vi "file.tif.Write.vi"(7 "name":string, 8 "error in":errorcluster, 10 "u16 pixmap":u16[][](array[numeric]), 11 "path":path) -> (0 "error out":errorcluster)   [LabVIEW 2020]
uses:
  lib/fileIO.x64.dll
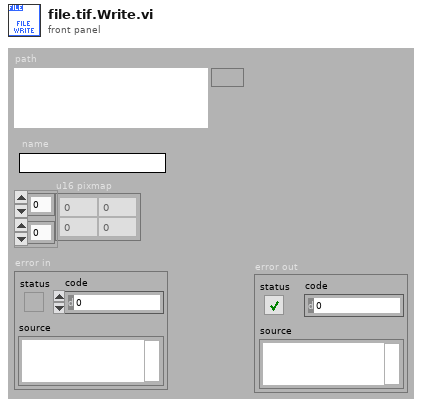
[diagram p1: front panel]
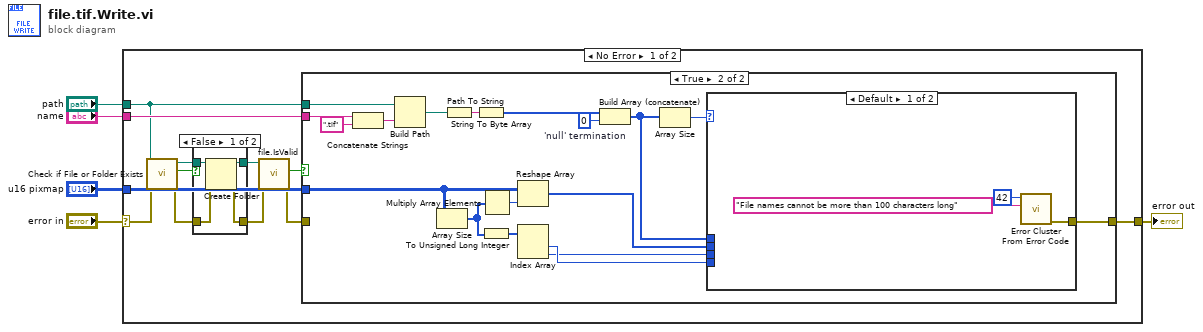
[diagram p0: block diagram]
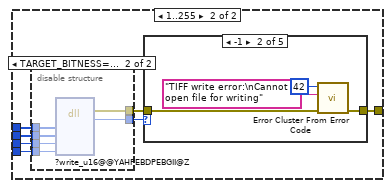
[diagram p3: hidden frame]
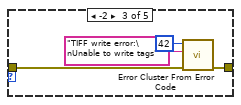
[diagram p5: hidden frame]
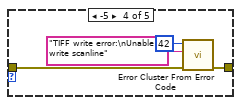
[diagram p6: hidden frame]
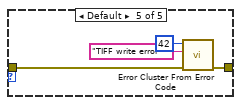
[diagram p7: hidden frame]
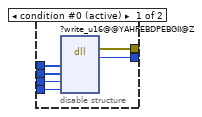
[diagram p8: hidden frame]
diagram:
  n1 = case shown="No Error" "error in" {
    selector: "error in" -> [w15 w82]
    tunnel: "path" -> [w6 _]
    tunnel: "u16 pixmap" -> [w17 _]
    tunnel: [w16 w82] -> w2
    tunnel: "name" -> [w9 _]
    frame No Error {
      n2 = call <vilib>:"Check if File or Folder Exists.vi"("error in (no error)"=w15, "path"=w6) -> ("error out"=w13:errorcluster, "file or folder exists?"=w11:bool, "dup path"=w7:path)  [unwired: 7 in]
      n3 = case shown="False" w11 {
        tunnel: w7 -> [w79 w80]
        tunnel: w13 -> [w78 w81]
        tunnel: [w77 w81] -> w12
        tunnel: [w76 w80] -> w8
        frame False {
          n4 = Create Folder(path (use dialog)=w79, error in=w78) -> (created path=w76:path, error out=w77:errorcluster)  [unwired: 1 in, 1 out]
        }
        frame True {
        }
      }
      n5 = call "file.IsValid.vi"("error in (no error)"=w12, "path"=w8) -> ("error out"=w14:errorcluster, "valid file/folder?"=w10:bool)  [unwired: 7 in, 1 out]
      n6 = case shown="True" w10 {
        tunnel: w17 -> [_ w21]
        tunnel: [w18 w26] -> w16
        tunnel: w14 -> [w18 _]
        tunnel: w6 -> [_ w22]
        tunnel: w9 -> [_ w23]
        frame False {
        }
        frame True {
          w34 = u8 0  # 'null' termination
          n7 = Concatenate Strings(w23, ".tif" ("string")) -> (w25:string)
          n8 = Build Path(base path=w22, name or relative path=w25) -> (appended path=w27:path)
          n9 = Array Size(array=w21) -> (size(s)=w32:i32[])
          n10 = Path To String(path=w27) -> (string=w29:string)
          n11 = String To Byte Array(string=w29) -> (unsigned byte array=w35:u8[])
          n12 = To Unsigned Long Integer(number=w32) -> (unsigned 32bit integer=w28:u32[])
          n13 = Multiply Array Elements(1:w32) -> (0:w33:i32)
          n14 = Reshape Array(w21, w33) -> (w36:u16[])
          n15 = Index Array(array=w28) -> (element #1=w31:u32, element #2=w30:u32)  [unwired: 2 in]
          n16 = Build Array (concatenate)(w35, w34) -> (w20:u8[])
          n17 = Array Size(array=w20) -> (size(s)=w19:i32)
          n18 = case shown="Default" w19 {
            tunnel: w36 -> [_ w46]
            tunnel: w31 -> [_ w45]
            tunnel: w30 -> [_ w44]
            tunnel: [w39 w41] -> w26
            tunnel: w20 -> [_ w40]
            frame Default {
              n19 = call <vilib>:"Error Cluster From Error Code.vi"("error message (\"\")"="File names cannot be more than 100 characters long" ("error message (\"\")"), "error code (0)"=42) -> ("error out"=w39:errorcluster)  [unwired: 7 in]
            }
            frame 1..255 {
              n20 = disable-structure shown="TARGET_BITNESS==32" {
                disable-tunnel: w46 -> [w69 w75]
                disable-tunnel: w45 -> [w68 w74]
                disable-tunnel: w44 -> [w67 w73]
                disable-tunnel: w40 -> [w66 w72]
                disable-tunnel: [w65 w71] -> w43
                disable-tunnel: [w64 w70] -> w42
                frame condition #0 (active) {
                  n21 = dll-call lib="C:/Users/pittsburger.SOLARIS/Desktop/UNSW/Solar Inspection System/v7/v0.7.5/lib/fileIO.x64.dll" fn="?write_u16@@YAHPEBDPEBGII@Z" label="write_u16"("szFilename"=w66, "pImageBuf"=w69, "width"=w67, "height"=w68) -> (error out=w64:errorcluster, "return type"=w65:i32)  [unwired: 7 in, 1 out]
                }
                frame condition #1 {
                  n22 = dll-call lib="C:/Users/pittsburger.SOLARIS/Desktop/UNSW/Solar Inspection System/v7/v0.7.5/lib/fileIO.x64.dll" fn="?write_u16@@YAHPEBDPEBGII@Z" label="write_u16"("szFilename"=w72, "pImageBuf"=w75, "width"=w73, "height"=w74) -> (error out=w70:errorcluster, "return type"=w71:i32)  [unwired: 7 in, 1 out]
                }
              }
              n23 = case shown="-1" w43 {
                tunnel: w42 -> [w47 w51 w55 w59 w63]
                tunnel: [w47 w50 w54 w58 w62] -> w41
                frame 0 {
                  # "No error"
                }
                frame -1 {
                  n24 = call <vilib>:"Error Cluster From Error Code.vi"("error in (no error)"=w51, "error message (\"\")"="TIFF write error:\nCannot open file for writing" ("error message (\"\")"), "error code (0)"=42) -> ("error out"=w50:errorcluster)  [unwired: 6 in]
                }
                frame -2 {
                  n25 = call <vilib>:"Error Cluster From Error Code.vi"("error in (no error)"=w55, "error message (\"\")"="TIFF write error:\nUnable to write tags" ("error message (\"\")"), "error code (0)"=42) -> ("error out"=w54:errorcluster)  [unwired: 6 in]
                }
                frame -5 {
                  n26 = call <vilib>:"Error Cluster From Error Code.vi"("error in (no error)"=w59, "error message (\"\")"="TIFF write error:\nUnable to write scanline" ("error message (\"\")"), "error code (0)"=42) -> ("error out"=w58:errorcluster)  [unwired: 6 in]
                }
                frame Default {
                  n27 = call <vilib>:"Error Cluster From Error Code.vi"("error in (no error)"=w63, "error message (\"\")"="TIFF write error" ("error message (\"\")"), "error code (0)"=42) -> ("error out"=w62:errorcluster)  [unwired: 6 in]
                }
              }
            }
          }
        }
      }
    }
    frame Error {
    }
  }
  "error out" <- w2
